vi "get_zoom.vi"(8 "error in (no error)":errorcluster, 11 "TrajectoryMG100122GenericFPGA in":refnum<class "TrajectoryMG100122GenericFPGA.lvclass">) -> (0 "error out":errorcluster, 2 "zoom":dbl, 3 "TrajectoryMG100122GenericFPGA out":refnum<class "TrajectoryMG100122GenericFPGA.lvclass">)   [LabVIEW 2010, in "TrajectoryMG100122GenericFPGA.lvclass"]
uses:
  TrajectoryMG100122GenericFPGA.lvclass
  TrajectoryMG100122GenericFPGA.lvclass/TrajectoryMG100122GenericFPGA.ctl
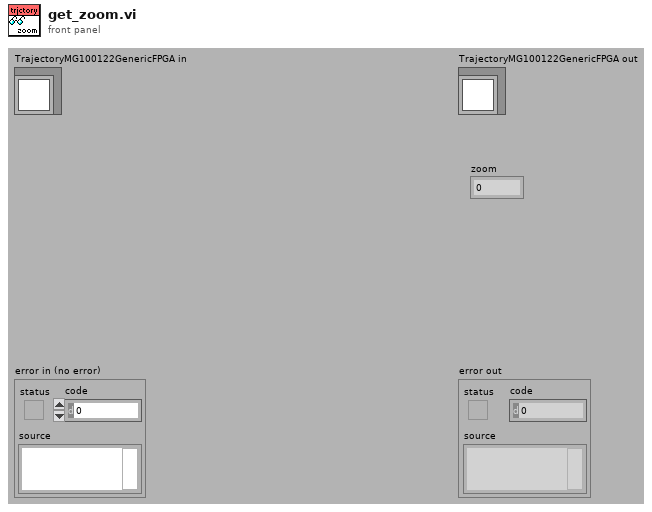
[diagram p1: front panel]
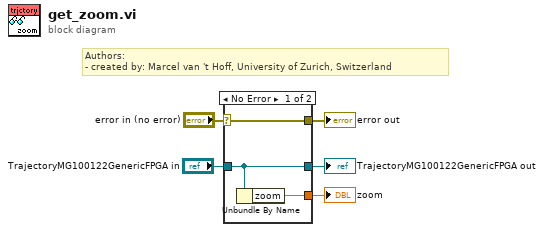
[diagram p0: block diagram]
diagram:
  # "Authors: \n- created by: Marcel van 't Hoff, University of Zurich, Switzerland"
  n1 = case shown="No Error" "error in (no error)" {
    selector: "error in (no error)" -> [w8 w10]
    tunnel: [w8 w10] -> w4
    tunnel: [w7 w9] -> w2
    tunnel: "TrajectoryMG100122GenericFPGA in" -> [w7 w9]
    tunnel: [w6 _] -> w1
    frame No Error {
      n2 = Unbundle By Name(w7) -> ("zoom"=w6:dbl)
    }
    frame Error {
    }
  }
  "error out" <- w4
  "TrajectoryMG100122GenericFPGA out" <- w2
  "zoom" <- w1
